vi "Speed Measurement Test.vi"() -> ()   [LabVIEW 2009]
uses:
  <vilib>/eio/EIONode/EIONode.xnode
  <vilib>/rvi/eio/nirviEIOImplementation/nirviEIOImplementation.xnode
  <vilib>/rvi/eio/common/nirviEmuTemplateMethod_noerrors.vi
  <vilib>/rvi/eio/common/nirviEmuClasses.ctl
panel:
  out "Drive Encoder Delta (ticks)":u32
  out "Drive Motor Speed (cpt)":fxp<+/-,20,1>
  out "The Steering Encoder Changed":bool
  out "Current Steering Encoder Value":i32
  out "Maximum Steering Encoder Count":i32
  out "Minimum Steering Encoder Count":i32
  out "The Lidar Encoder Changed":bool
  out "Current Lidar Encoder Value":i32
  out "Maximum Lidar Encoder Count":i32
  out "Minimum Lidar Encoder Count":i32
  out "Minimum Drive Encoder Count":i32
  out "Maximum Drive Encoder Count":i32
  out "Current Drive Encoder Value":i32
  out "The Drive Encoder Changed":bool
  out "Steering Encoder A":bool
  out "Steering Encoder B":bool
  out "Steering Encoder Index":bool
  out "Lidar Encoder A":bool
  out "Lidar Encoder B":bool
  out "Lidar Encoder Index":bool
  out "Drive Encoder A":bool
  out "Drive Encoder B":bool
  out "Drive Encoder Index":bool
  in  "stop":bool
  in  "Lidar Enable":bool
  in  "Steering Enable":bool
  in  "Drive Enable":bool
  in  "Lidar output Voltage":fxp<+/-,20,5>
  in  "Steering output Voltage":fxp<+/-,20,5>
  in  "Drive output Voltage":fxp<+/-,20,5>
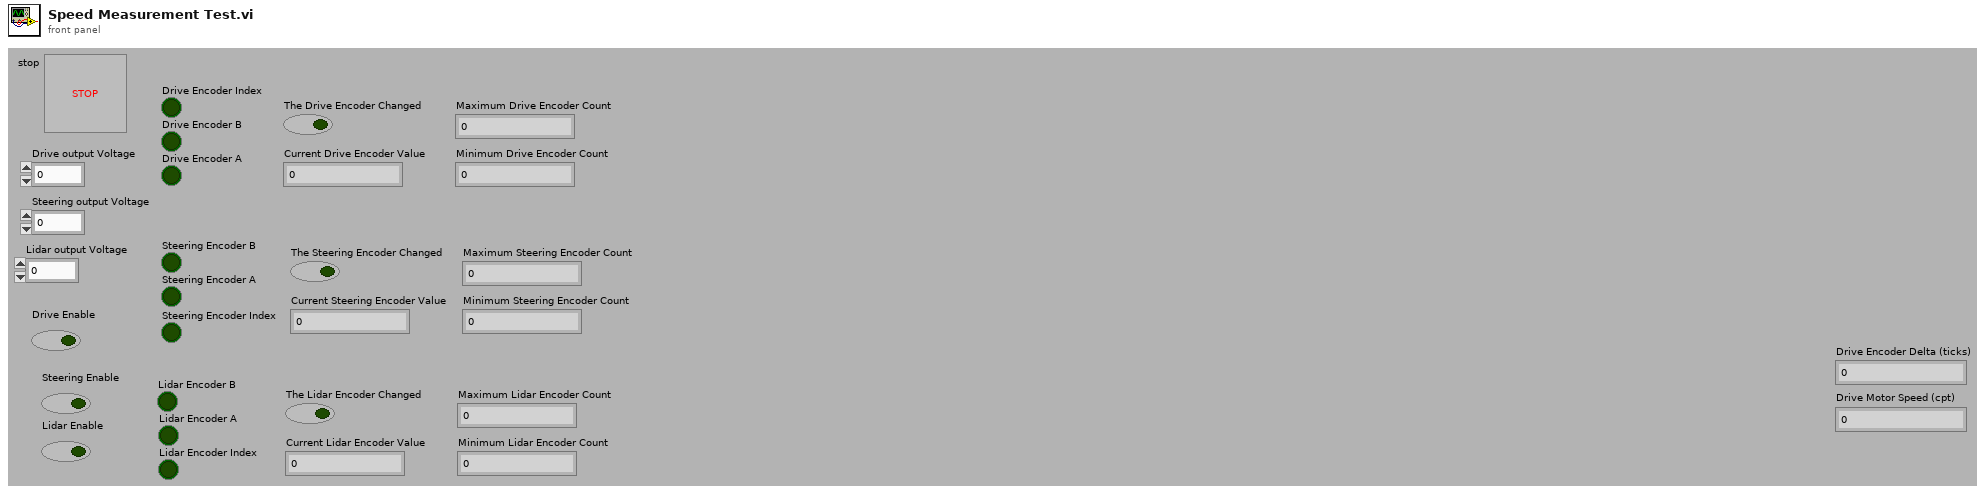
[diagram p1: front panel]
types:
  T1 = typedef "nirviEmuClasses.ctl" = enum16{"IO Read", "IO Write", "Method", "Property Read", "Property Write"}
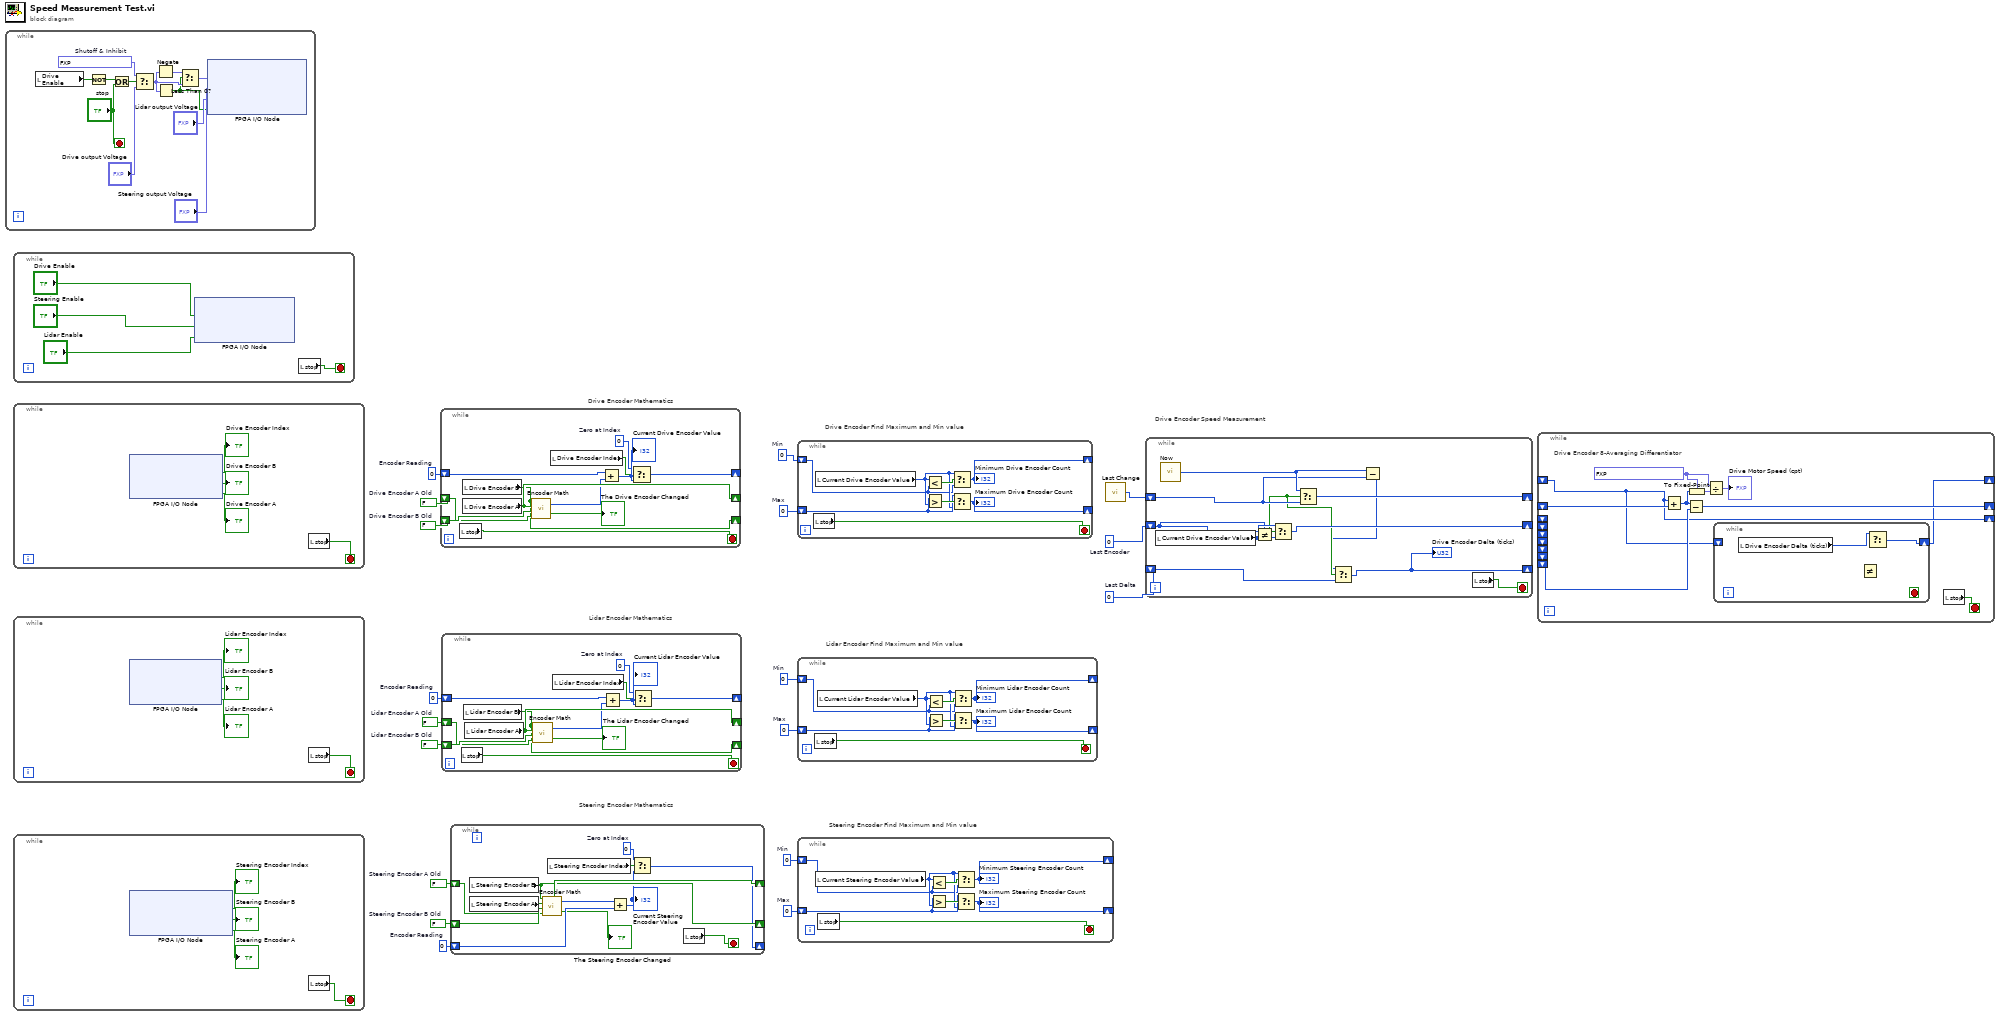
[diagram p0: block diagram]
diagram:
  w1 = u32 0  # Last Delta
  w2 = 0  # Last Encoder
  w4 = 0  # Min
  w5 = 0  # Max
  w6 = 0  # Encoder Reading
  w7 = FALSE  # Steering Encoder A Old
  w8 = FALSE  # Steering Encoder B Old
  w13 = 0  # Min
  w12 = 0  # Max
  w11 = 0  # Encoder Reading
  w10 = FALSE  # Lidar Encoder A Old
  w9 = FALSE  # Lidar Encoder B Old
  w14 = 0  # Min
  w15 = 0  # Max
  w16 = 0  # Encoder Reading
  w17 = FALSE  # Drive Encoder A Old
  w18 = FALSE  # Drive Encoder B Old
  # "Drive Encoder Speed Measurement"
  # "Steering Encoder Find Maximum and Min value"
  # "Steering Encoder Mathematics"
  # "Lidar Encoder Find Maximum and Min value"
  # "Lidar Encoder Mathematics"
  # "Drive Encoder Find Maximum and Min value"
  # "Drive Encoder Mathematics"
  n1 = while {
    stop <- "stop" stop-if-true
    w27 = fxp<+/-,20,5> 0.0  # Shutoff & Inhibit
    n2 = local read "Drive Enable"() -> (w25:bool)
    n3 = Not(x=w25) -> (.not. x?=w24:bool)
    n4 = Or(x=w24, y="stop") -> (x .or. y?=w23:bool)
    n5 = Select(t=w27, s=w23, f="Drive output Voltage") -> (s? t:f=w21:fxp<+/-,20,5>)
    n6 = Negate(x=w21) -> (-x=w20:fxp<+/-,20,5>)
    n7 = Less Than 0?(x=w21) -> (x < 0?=w19:bool)
    n8 = Select(t=w20, s=w19, f=w21) -> (s? t:f=w22:fxp<+/-,20,5>)
    n9 = xnode "FPGA I/O Node"("Drive Motor Speed"=w22, "Steering Motor Speed"="Steering output Voltage", "Lidar Motor Speed"="Lidar output Voltage", "Drive Motor Reverse"=w19) -> ()  [unwired: 4 in, 4 out]
  }
  n10 = while {
    stop <- w75 stop-if-true
    n11 = xnode "FPGA I/O Node"("Drive Motor Enable"="Drive Enable", "Steering Motor Inhibit"="Steering Enable", "Lidar Motor Inhibit"="Lidar Enable") -> ()  [unwired: 3 in, 3 out]
    n12 = local read "stop"() -> (w75:bool)
  }
  n13 = while {
    stop <- w115 stop-if-true
    n14 = xnode "FPGA I/O Node"() -> ("Drive Encoder Index"=→"Drive Encoder Index":bool, "Drive Encoder B"=→"Drive Encoder B":bool, "Drive Encoder A"=→"Drive Encoder A":bool)  [unwired: 3 in, 3 out]
    n15 = local read "stop"() -> (w115:bool)
  }
  n16 = while {
    stop <- w176 stop-if-true
    n17 = xnode "FPGA I/O Node"() -> ("Lidar Encoder Index"=→"Lidar Encoder Index":bool, "Lidar Encoder B"=→"Lidar Encoder B":bool, "Lidar Encoder A"=→"Lidar Encoder A":bool)  [unwired: 3 in, 3 out]
    n18 = local read "stop"() -> (w176:bool)
  }
  n19 = while {
    stop <- w237 stop-if-true
    n20 = xnode "FPGA I/O Node"() -> ("Steering Encoder Index"=→"Steering Encoder Index":bool, "Steering Encoder B"=→"Steering Encoder B":bool, "Steering Encoder A"=→"Steering Encoder A":bool)  [unwired: 3 in, 3 out]
    n21 = local read "stop"() -> (w237:bool)
  }
  n22 = while {
    shift-right: [w304] -> _
    shift-left: w17 -> [w305]
    shift-right: [w303] -> _
    shift-left: w18 -> [w306]
    shift-right: [w298] -> _
    shift-left: w16 -> [w302]
    stop <- w295 stop-if-true
    w296 = 0  # Zero at Index
    n23 = local read "stop"() -> (w295:bool)
    n24 = local read "Drive Encoder B"() -> (w303:bool)
    n25 = local read "Drive Encoder A"() -> (w304:bool)
    n26 = call "Encoder Math.vi"("Encoder A_old"=w305, "Encoder B_old"=w306, "Encoder A_new"=w304, "Encoder B_new"=w303) -> ("The Encoder Changed"=→"The Drive Encoder Changed":bool, "Change in Encoder Value"=w301:i32)
    n27 = local read "Drive Encoder Index"() -> (w297:bool)
    n28 = Add(x=w302, y=w301) -> (x+y=w299:i32)
    "Current Drive Encoder Value" <- w299
    n29 = Select(t=w296, s=w297, f=w299) -> (s? t:f=w298:i32)
  }
  n30 = while {
    shift-right: [w316] -> _
    shift-left: w10 -> [w317]
    shift-right: [w315] -> _
    shift-left: w9 -> [w318]
    shift-right: [w310] -> _
    shift-left: w11 -> [w314]
    stop <- w307 stop-if-true
    w308 = 0  # Zero at Index
    n31 = local read "stop"() -> (w307:bool)
    n32 = local read "Lidar Encoder B"() -> (w315:bool)
    n33 = local read "Lidar Encoder A"() -> (w316:bool)
    n34 = call "Encoder Math.vi"("Encoder A_old"=w317, "Encoder B_old"=w318, "Encoder A_new"=w316, "Encoder B_new"=w315) -> ("The Encoder Changed"=→"The Lidar Encoder Changed":bool, "Change in Encoder Value"=w313:i32)
    n35 = local read "Lidar Encoder Index"() -> (w309:bool)
    n36 = Add(x=w314, y=w313) -> (x+y=w311:i32)
    "Current Lidar Encoder Value" <- w311
    n37 = Select(t=w308, s=w309, f=w311) -> (s? t:f=w310:i32)
  }
  n38 = while {
    shift-right: [w328] -> _
    shift-left: w7 -> [w329]
    shift-right: [w327] -> _
    shift-left: w8 -> [w330]
    shift-right: [w322] -> _
    shift-left: w6 -> [w326]
    stop <- w319 stop-if-true
    w320 = 0  # Zero at Index
    n39 = local read "Steering Encoder B"() -> (w327:bool)
    n40 = local read "Steering Encoder A"() -> (w328:bool)
    n41 = call "Encoder Math.vi"("Encoder A_old"=w329, "Encoder B_old"=w330, "Encoder A_new"=w328, "Encoder B_new"=w327) -> ("The Encoder Changed"=→"The Steering Encoder Changed":bool, "Change in Encoder Value"=w325:i32)
    n42 = local read "Steering Encoder Index"() -> (w321:bool)
    n43 = Add(x=w325, y=w326) -> (x+y=w323:i32)
    "Current Steering Encoder Value" <- w323
    n44 = Select(t=w320, s=w321, f=w323) -> (s? t:f=w322:i32)
    n45 = local read "stop"() -> (w319:bool)
  }
  n46 = while {
    shift-right: [w336] -> _
    shift-left: w15 -> [w337]
    shift-right: [w332] -> _
    shift-left: w14 -> [w333]
    stop <- w331 stop-if-true
    n47 = local read "stop"() -> (w331:bool)
    n48 = local read "Current Drive Encoder Value"() -> (w334:i32)
    n49 = Less?(x=w334, y=w333) -> (x < y?=w335:bool)
    n50 = Greater?(x=w337, y=w334) -> (0:w338:bool)
    n51 = Select(t=w334, s=w335, f=w333) -> (s? t:f=w332:i32)
    "Minimum Drive Encoder Count" <- w332
    n52 = Select(t=w337, s=w338, f=w334) -> (s? t:f=w336:i32)
    "Maximum Drive Encoder Count" <- w336
  }
  n53 = while {
    shift-right: [w344] -> _
    shift-left: w12 -> [w345]
    shift-right: [w340] -> _
    shift-left: w13 -> [w341]
    stop <- w339 stop-if-true
    n54 = local read "stop"() -> (w339:bool)
    n55 = local read "Current Lidar Encoder Value"() -> (w342:i32)
    n56 = Less?(x=w342, y=w341) -> (x < y?=w343:bool)
    n57 = Greater?(x=w345, y=w342) -> (0:w346:bool)
    n58 = Select(t=w342, s=w343, f=w341) -> (s? t:f=w340:i32)
    "Minimum Lidar Encoder Count" <- w340
    n59 = Select(t=w345, s=w346, f=w342) -> (s? t:f=w344:i32)
    "Maximum Lidar Encoder Count" <- w344
  }
  n60 = while {
    shift-right: [w352] -> _
    shift-left: w5 -> [w353]
    shift-right: [w348] -> _
    shift-left: w4 -> [w349]
    stop <- w347 stop-if-true
    n61 = local read "Current Steering Encoder Value"() -> (w350:i32)
    n62 = local read "stop"() -> (w347:bool)
    n63 = Less?(x=w350, y=w349) -> (x < y?=w351:bool)
    n64 = Greater?(x=w353, y=w350) -> (0:w354:bool)
    n65 = Select(t=w350, s=w351, f=w349) -> (s? t:f=w348:i32)
    "Minimum Steering Encoder Count" <- w348
    n66 = Select(t=w353, s=w354, f=w350) -> (s? t:f=w352:i32)
    "Maximum Steering Encoder Count" <- w352
  }
  n67 = call "Last Change"() -> ("Tick Count(Ticks)"=w3:u32)
  n68 = while {
    shift-right: [w362] -> _
    shift-left: w3 -> [w360]
    shift-right: [w363] -> _
    shift-left: w2 -> [w364]
    shift-right: [w356] -> _
    shift-left: w1 -> [w357]
    stop <- w355 stop-if-true
    n69 = local read "Current Drive Encoder Value"() -> (w365:i32)
    n70 = call "Now"() -> ("Tick Count(Ticks)"=w361:u32)
    n71 = Not Equal?(x=w364, y=w365) -> (x != y?=w359:bool)
    n72 = Select(t=w365, s=w359, f=w364) -> (s? t:f=w363:i32)
    n73 = Select(t=w361, s=w359, f=w360) -> (s? t:f=w362:u32)
    n74 = Subtract(x=w361, y=w360) -> (x-y=w358:u32)
    n75 = Select(t=w358, s=w359, f=w357) -> (s? t:f=w356:u32)
    "Drive Encoder Delta (ticks)" <- w356
    n76 = local read "stop"() -> (w355:bool)
  }
  n77 = while {
    shift-right: [w371] -> _
    shift-left: _ -> [w370]
    shift-right: [w367] -> _
    shift-left: _ -> [_]
    shift-left: _ -> [_]
    shift-left: _ -> [_]
    shift-left: _ -> [_]
    shift-left: _ -> [_]
    shift-left: _ -> [_]
    shift-left: _ -> [w369]
    shift-right: [w366] -> _
    shift-left: _ -> [w367]
    stop <- w373 stop-if-true
    w374 = fxp<+/-,32,32> 8.0 ("fixed-point type")
    # "Drive Encoder 8-Averaging Differentiator"
    n78 = Add(x=w367, y=w370) -> (x+y=w372:u32)
    n79 = Subtract(x=w372, y=w369) -> (x-y=w371:u32)
    n80 = To Fixed-Point(fixed-point type=w374, number=w372) -> (fixed-point=w375:fxp<+/-,32,32>)
    n81 = Divide(x=w374, y=w375) -> (x/y=→"Drive Motor Speed (cpt)":fxp<+/-,20,1>)
    n82 = while {
      shift-right: [w377] -> w366
      shift-left: w367 -> [_]
      stop <- _ stop-if-true
      n83 = local read "Drive Encoder Delta (ticks)"() -> (w376:u32)
      n84 = Not Equal?() -> ()  [unwired: 2 in, 1 out]
      n85 = Select(t=w376) -> (s? t:f=w377:u32)  [unwired: 2 in]
    }
    n86 = local read "stop"() -> (w373:bool)
  }
